vi "Close.vi"(8 "error in (no error)":errorcluster {"code" format="%.0x"}, 11 "VISA Resource Name":refnum<visa-resource-name>) -> (0 "error out":errorcluster {"code" format="%.0x"})   [LabVIEW 2010, in "Tektronix TDS 3000 Series.lvlib"]
doc: "Closes the I/O interface and returns the instrument to local mode."
uses:
  <instrlib>/Tektronix TDS 3000 Series/Tektronix TDS 3000 Series.lvlib
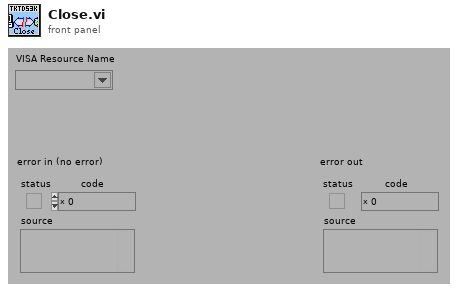
[diagram p1: front panel]
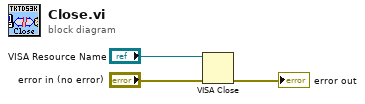
[diagram p0: block diagram]
diagram:
  n1 = VISA Close(VISA resource name="VISA Resource Name", error in (no error)="error in (no error)") -> (error out=→"error out":errorcluster)
